vi "Get Nearest Color Name.vi"(4 "Color to Match":u32(colorbox), 5 "Color Names & Values":T1) -> (0 "Name":string, 1 "Nearest Color":u32(colorbox))   [LabVIEW 2015, in "GraphViz Mapping Visualizer.lvlib"]
doc: "From Color Names and Values, finds the nearest color to match and its name."
uses:
  GraphViz Mapping Visualizer.lvlib
panel:
  out "Error":i16
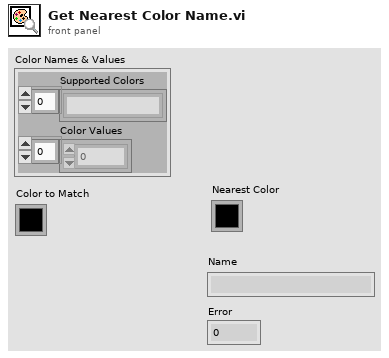
[diagram p1: front panel]
types:
  T1 = cluster{"Supported Colors":string[], "Color Values":u32[]}
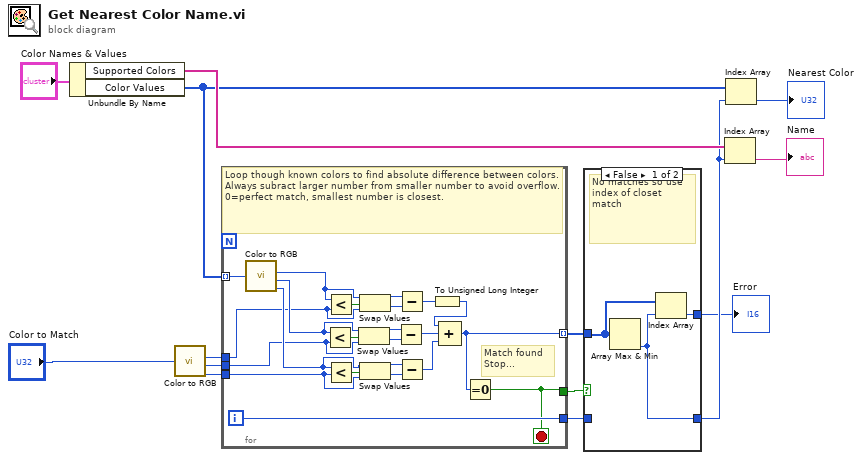
[diagram p0: block diagram]
diagram:
  n1 = Unbundle By Name("Color Names & Values") -> ("Supported Colors"=w13:string[], "Color Values"=w6:u32[])
  n2 = call <vilib>:"Color to RGB.vi"("Color"="Color to Match") -> ("R"=w9:u8, "G"=w8:u8, "B"=w7:u8)  [unwired: 1 out]
  n3 = for {
    tunnel: w9 -> [w17]
    tunnel: w8 -> [w20]
    tunnel: w7 -> [w22]
    tunnel: w6 -> [w37] mode=indexing
    tunnel: [w36] -> w4 mode=indexing
    tunnel: [w35] -> w3
    tunnel: [w34] -> w5
    i -> [w35]
    stop <- w34 stop-if-true
    # "Match found\nStop..."
    # "Loop though known colors to find absolute difference between colors. Always subract larger number from smaller number to avoid overflow. \n0=perfect match, smallest number is closest."
    n4 = call <vilib>:"Color to RGB.vi"("Color"=w37) -> ("R"=w18:u8, "G"=w19:u8, "B"=w21:u8)  [unwired: 1 out]
    n5 = Less?(x=w19, y=w20) -> (x < y?=w29:bool)
    n6 = Less?(x=w18, y=w17) -> (x < y?=w26:bool)
    n7 = Less?(x=w21, y=w22) -> (x < y?=w33:bool)
    n8 = Swap Values(12:w19, 13:w29, 14:w20) -> (1:w28:u8, 3:w27:u8)
    n9 = Swap Values(12:w18, 13:w26, 14:w17) -> (1:w25:u8, 3:w24:u8)
    n10 = Swap Values(12:w21, 13:w33, 14:w22) -> (1:w32:u8, 3:w31:u8)
    n11 = Subtract(x=w28, y=w27) -> (x-y=w23:u8)
    n12 = Subtract(x=w25, y=w24) -> (x-y=w16:u8)
    n13 = Subtract(x=w32, y=w31) -> (x-y=w30:u8)
    n14 = To Unsigned Long Integer(number=w16) -> (unsigned 32bit integer=w15:u32)
    n15 = Compound Arithmetic op=ADD(w15, w23, w30) -> (w36:u32)
    n16 = Equal To 0?(x=w36) -> (x = 0?=w34:bool)
  }
  n17 = case shown="False" w5 {
    tunnel: w4 -> [w40 _]
    tunnel: w3 -> [_ w41]
    tunnel: [w39 w41] -> w2
    tunnel: [w38 _] -> w1
    frame False {
      # "No matches so use index of closet match"
      n18 = Array Max & Min(array=w40) -> (min index (indices)=w39:i32)  [unwired: 3 out]
      n19 = Index Array(array=w40, index=w39) -> (element=w38:u32)
    }
    frame True {
      # "Got Match so use index \nof exact \nmatch."
    }
  }
  "Error" <- w1
  n20 = Index Array(array=w13, index=w2) -> (element=→"Name":string)
  n21 = Index Array(array=w6, index=w2) -> (element=→"Nearest Color":u32)
